vi "Write Time interval.vi"(8 "error in (no error)":errorcluster, 10 "Time interval":i64 caption="Time interval [µs]", 11 "Time in":refnum<class "Time.lvclass">) -> (0 "error out":errorcluster, 3 "Time out":refnum<class "Time.lvclass">)   [LabVIEW 2013, in "HardwareCharacterization.lvlib" / "Time.lvclass"]
uses:
  Time.lvclass
  Time.lvclass/Time.ctl
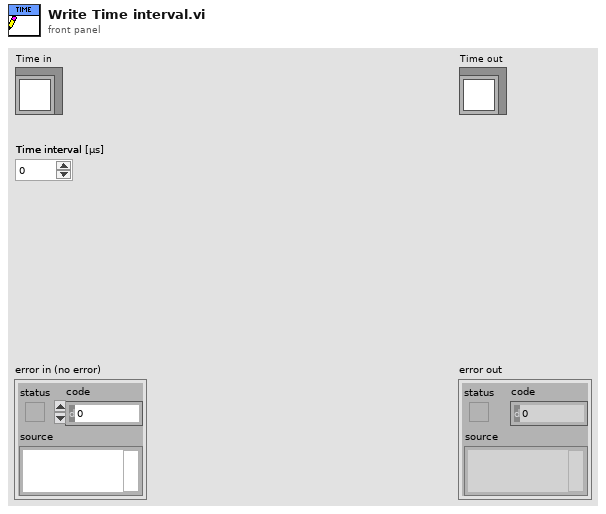
[diagram p1: front panel]
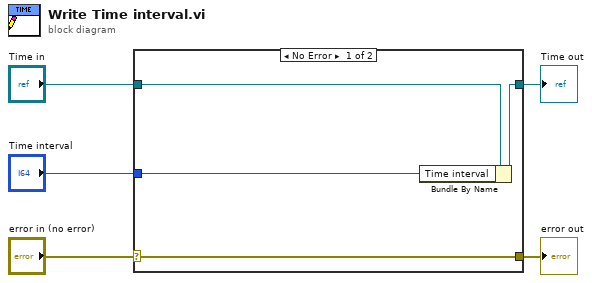
[diagram p0: block diagram]
diagram:
  n1 = case shown="No Error" "error in (no error)" {
    selector: "error in (no error)" -> [w9 w10]
    tunnel: [w9 w10] -> w4
    tunnel: [w7 w11] -> w2
    tunnel: "Time in" -> [w8 w11]
    tunnel: "Time interval" -> [w6 _]
    frame No Error {
      n2 = Bundle By Name(cluster=w8, "Time interval"=w6) -> (w7:refnum<class "Time.lvclass">)
    }
    frame Error {
    }
  }
  "error out" <- w4
  "Time out" <- w2
